vi "testing_delay_and_cw_sweep.vi"() -> ()   [LabVIEW 2015, in "Tausand AB1000.lvlib"]
uses:
  <instrlib>/Tausand AB1000/Tausand AB1000.lvlib
  <instrlib>/Tausand AB1000/Public/Controls/deviceTypeRing.ctl
  <instrlib>/Tausand AB1000/Public/Controls/channelRing.ctl
  <instrlib>/Tausand AB1000/Public/Controls/counters4ch.ctl
panel:
  out "i case":i32
  out "total cases":i32
  in  "Stop Button":bool
  out "coinc Chart":T1(graph)
  out "current values":T2
  out "delayed channel":T3 items=["none", "A", "B", "C", "D", "E", "F", "G", "H"]
  in  "sampling (ms)":u32=1000
  out "i delay":i32
  out "i ch":i32
  out "i cw":i32
  out "values":u32[][][][](array[numeric])
  out "device type":T4 items=["any"=0, "AB1002"=1002, "AB1004"=1004, "AB1502"=1502, "AB1504"=1504, "AB1902"=1902, "AB1904"=1904]
  out "cw array":u32[](array[numeric])
  out "delay array":u32[](array[numeric])
  in  "step cw":u32=1
  in  "max cw":u32=10
  in  "min cw":u32=1
  in  "step delay":u32=1
  in  "max delay":u32=20
  in  "min delay":u32
  out "current delay (ns)":u32
  out "current cw (ns)":u32
  in  "VISA resource name":refnum<visa-resource-name>
  # "case"
  # "out of"
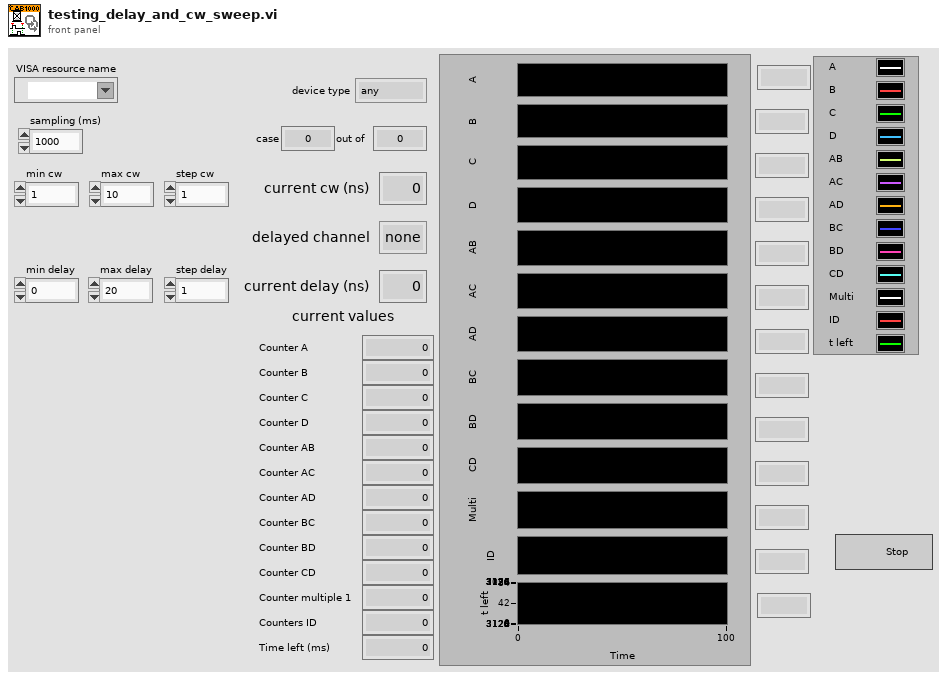
[diagram p1: front panel]
types:
  T1 = cluster{"counter_A":u32, "counter_B":u32, "counter_C":u32, "counter_D":u32, "counter_AB":u32, "counter_AC":u32, "counter_AD":u32, "counter_BC":u32, "counter_BD":u32, "counter_CD":u32, "counter_multiple_1":u32, "counters_ID":u32, "time_left":u32}
  T2 = typedef "Tausand AB1000.lvlib/counters4ch.ctl" = cluster{"counter_A":u32, "counter_B":u32, "counter_C":u32, "counter_D":u32, "counter_AB":u32, "counter_AC":u32, "counter_AD":u32, "counter_BC":u32, "counter_BD":u32, "counter_CD":u32, "counter_multiple_1":u32, "counters_ID":u32, "time_left":u32}
  T3 = typedef "Tausand AB1000.lvlib/channelRing.ctl" = u8
  T4 = typedef "Tausand AB1000.lvlib/deviceTypeRing.ctl" = u16
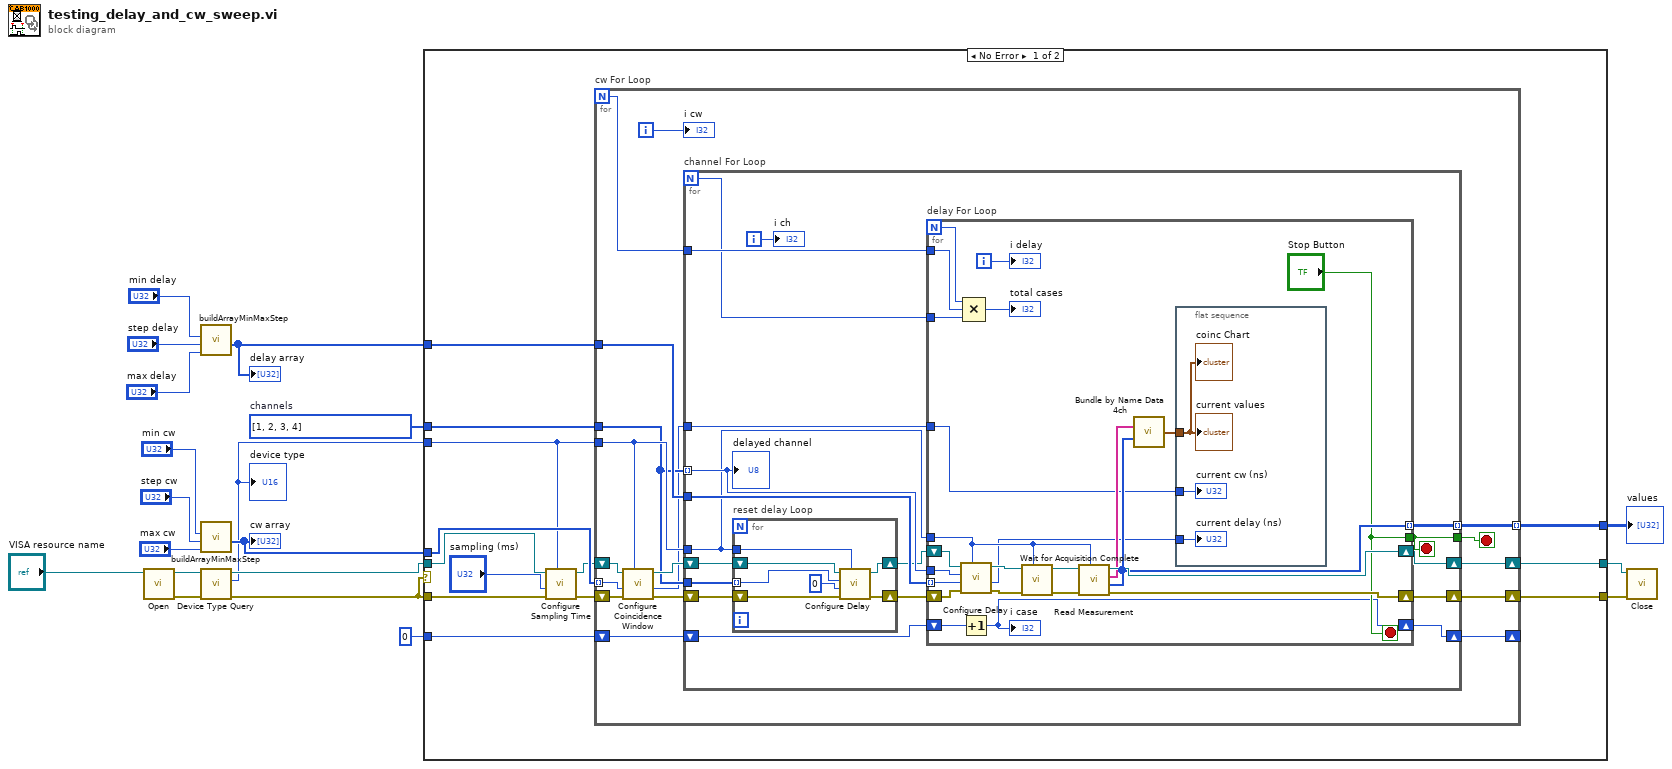
[diagram p0: block diagram]
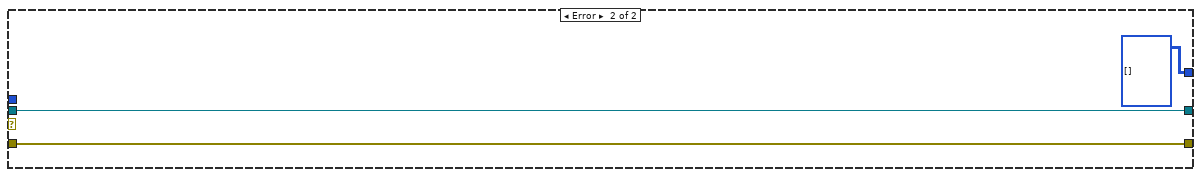
[diagram p2: hidden frame]
diagram:
  w6 = T3[] [1, 2, 3, 4] items=["none", "A", "B", "C", "D", "E", "F", "G", "H"]  # channels
  n1 = call <instrlib>:"Open.vi"("VISA resource name"="VISA resource name") -> ("error out"=w11:errorcluster, "VISA resource name out"=w10:refnum<visa-resource-name>)  [unwired: 9 in]
  n2 = call <instrlib>:"buildArrayMinMaxStep.vi"("max (10)"="max delay", "step (1)"="step delay", "min (0)"="min delay") -> ("array"=w7:i32[])  [unwired: 8 in]
  "delay array" <- w7
  n3 = call <instrlib>:"buildArrayMinMaxStep.vi"("max (10)"="max cw", "step (1)"="step cw", "min (0)"="min cw") -> ("array"=w12:i32[])  [unwired: 8 in]
  "cw array" <- w12
  n4 = call <instrlib>:"Device Type Query.vi"("error in (no error)"=w11, "VISA Refnum in"=w10) -> ("error out"=w2:errorcluster, "device type"=w8:T4, "VISA Refnum out"=w9:refnum<visa-resource-name>)  [unwired: 7 in]
  "device type" <- w8
  n5 = case shown="No Error" w2 {
    tunnel: w12 -> [w32 _]
    tunnel: w2 -> [w25 w104]
    tunnel: w9 -> [w26 w103]
    tunnel: w8 -> [w24 _]
    tunnel: w7 -> [w31 _]
    tunnel: w6 -> [w27 _]
    tunnel: [w30 u32[][][][] [] ("values")] -> w5
    tunnel: [w29 w103] -> w4
    tunnel: [w28 w104] -> w3
    tunnel: 0 ("i delay") -> [w20 _]
    frame No Error {
      n6 = call <instrlib>:"Configure Sampling Time.vi"("device type"=w24, "error in (no error)"=w25, "value (1000 ms)"="sampling (ms)", "VISA Refnum in"=w26) -> ("error out"=w22:errorcluster, "VISA Refnum out"=w21:refnum<visa-resource-name>)  [unwired: 5 in, 1 out]
      n7 = for "cw For Loop" {
        N -> [w37]
        tunnel: w32 -> [w47] mode=indexing
        tunnel: w24 -> [w43]
        tunnel: w31 -> [w46]
        tunnel: w27 -> [w39]
        tunnel: [w42] -> w30 mode=indexing
        shift-right: [w41] -> w28
        shift-left: w22 -> [w48]
        shift-right: [w40] -> w29
        shift-left: w21 -> [w49]
        shift-right: [w34] -> _
        shift-left: w20 -> [w35]
        i -> [w36]
        stop <- w38 stop-if-true
        n8 = call <instrlib>:"Configure Coincidence Window.vi"("device type"=w43, "error in (no error)"=w48, "value ns (10ns)"=w47, "VISA Refnum in"=w49) -> ("error out"=w44:errorcluster, "value ns out"=w33:u32, "VISA Refnum out"=w45:refnum<visa-resource-name>)  [unwired: 5 in]
        n9 = for "channel For Loop" {
          N -> [w54]
          tunnel: w46 -> [w67]
          tunnel: w43 -> [w57]
          tunnel: w39 -> [w66] mode=indexing
          tunnel: [w65] -> w42 mode=indexing
          shift-right: [w64] -> w41
          shift-left: w44 -> [w62]
          shift-right: [w63] -> w40
          shift-left: w45 -> [w61]
          tunnel: w39 -> [w58]
          tunnel: [w56] -> w38
          tunnel: w37 -> [w55]
          shift-right: [w51] -> w34
          shift-left: w35 -> [w52]
          tunnel: w33 -> [w50]
          i -> [w53]
          stop <- w56 stop-if-true
          n10 = for "reset delay Loop" {
            tunnel: w58 -> [w73] mode=indexing
            tunnel: w57 -> [w71]
            shift-right: [w69] -> w59
            shift-left: w62 -> [w70]
            shift-right: [w68] -> w60
            shift-left: w61 -> [w74]
            n11 = call <instrlib>:"Configure Delay.vi"("device type"=w71, "error in (no error)"=w70, "value (0 ns)"=u32 0, "channel"=w73, "VISA Refnum in"=w74) -> ("error out"=w69:errorcluster, "VISA Refnum out"=w68:refnum<visa-resource-name>)  [unwired: 4 in, 1 out]
          }
          n12 = for "delay For Loop" {
            N -> [w79]
            tunnel: w67 -> [w98] mode=indexing
            tunnel: w57 -> [w88]
            tunnel: w66 -> [w95]
            tunnel: [w86] -> w65 mode=indexing
            shift-right: [w94] -> w64
            shift-left: w59 -> [w96]
            shift-right: [w93] -> w63
            shift-left: w60 -> [w97]
            tunnel: ["Stop Button"] -> w56
            tunnel: w55 -> [w78]
            tunnel: w54 -> [w77]
            shift-right: [w80] -> w51
            shift-left: w52 -> [w81]
            tunnel: w50 -> [w75]
            i -> [w82]
            stop <- "Stop Button" stop-if-true
            n13 = call <instrlib>:"Configure Delay.vi"("device type"=w88, "error in (no error)"=w96, "value (0 ns)"=w98, "channel"=w95, "VISA Refnum in"=w97) -> ("error out"=w92:errorcluster, "value ns out"=w76:u32, "VISA Refnum out"=w90:refnum<visa-resource-name>)  [unwired: 4 in]
            n14 = Increment(x=w81) -> (x+1=w80:i32)
            "i case" <- w80
            n15 = Compound Arithmetic op=MULTIPLY(w79, w78, w77) -> (→"total cases":i32)
            n16 = call <instrlib>:"Wait for Acquisition Complete.vi"("device type"=w88, "error in (no error)"=w92, "VISA resource name"=w90) -> ("error out"=w91:errorcluster, "VISA resource name out"=w89:refnum<visa-resource-name>)  [unwired: 7 in]
            n17 = call <instrlib>:"Read Measurement.vi"("device type"=w88, "error in (no error)"=w91, "VISA Refnum in"=w89) -> ("error out"=w94:errorcluster, "values"=w86:u32[], "labels"=w87:string[], "VISA Refnum out"=w93:refnum<visa-resource-name>)  [unwired: 3 in, 2 out]
            n18 = call <instrlib>:"Bundle by Name Data 4ch.vi"("names"=w87, "values"=w86) -> ("output cluster 4ch"=w85:T2)  [unwired: 13 in]
            n19 = flat-sequence {
              tunnel: w85 -> [w101]
              tunnel: w76 -> [w100]
              tunnel: w75 -> [w99]
              frame #0 {
                "current values" <- w101
                "coinc Chart" <- w101
                "current delay (ns)" <- w100
                "current cw (ns)" <- w99
              }
            }
            "i delay" <- w82
          }
          "i ch" <- w53
          "delayed channel" <- w66
        }
        "i cw" <- w36
      }
    }
    frame Error {
    }
  }
  "values" <- w5
  n20 = call <instrlib>:"Close.vi"("error in (no error)"=w3, "VISA resource name"=w4) -> ()  [unwired: 9 in, 1 out]
